vi "Result_Test.vi"(8 "error in (no error)":errorcluster caption="entrée d'erreur (pas d'erreur)", 11 "Get_Voltage en ent rée":refnum<class "Zigbee_Start_Permit_Join.lvclass">) -> (0 "error out":errorcluster caption="sortie d'erreur", 3 "Get_Voltage en sortie":refnum<class "Zigbee_Start_Permit_Join.lvclass">)   [LabVIEW 2020, in "Library Test.lvlib" / "Zigbee_Start_Permit_Join.lvclass"]
uses:
  Zigbee_Start_Permit_Join.lvclass
  C:/Users/ngarcin/OneDrive - Altyor/Standard TB/Suite TB45/Class/Test/Test (Default)/Test (Default).lvclass
  C:/Users/ngarcin/OneDrive - Altyor/Standard TB/Suite TB45/Class/Test/Zigbee_Send_Command_UART/Zigbee_Send_Command_UART.lvclass
  Commun VI/TypeDef/Variable Printable.ctl
  Zigbee_Send_Command_UART/Zigbee_Send_Command_UART.lvclass
  Commun VI/Library Commun.lvlib
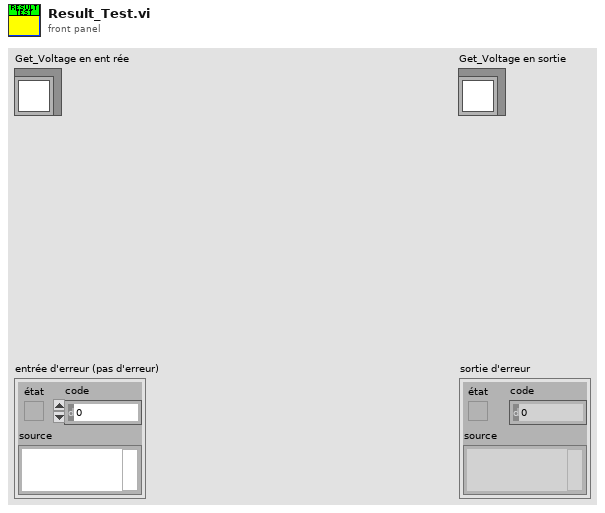
[diagram p1: front panel]
types:
  T1 = typedef "Variable Printable.ctl" = string
  T2 = enum16{"Get Variable", "Get All Variables", "Set Variable", "Delete Variable", "Delete All Variable"}
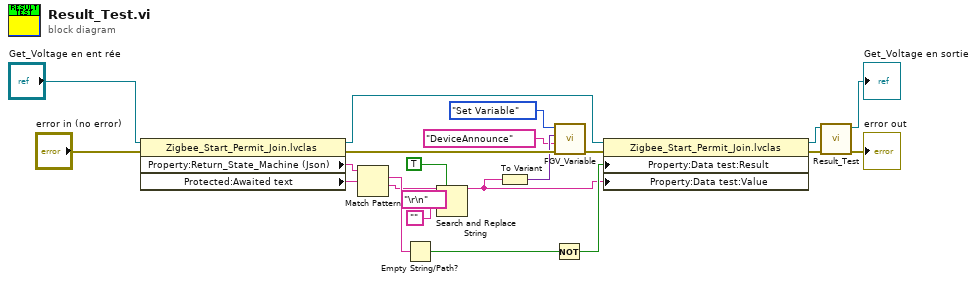
[diagram p0: block diagram]
diagram:
  n1 = property class="Zigbee_Start_Permit_Join.lvclas"(reference="Get_Voltage en ent rée", error in="error in (no error)") -> (reference out=w20:refnum<class "Zigbee_Start_Permit_Join.lvclass">, error out=w18:errorcluster, "Property:Return_State_Machine (Json)"=w17:string, "Protected:Awaited text"=w16:string)
  n2 = Match Pattern(string=w17, regular expression=w16) -> (match substring=w8:string, after substring=w4:string)  [unwired: 1 in, 2 out]
  n3 = Empty String/Path?(string/path=w8) -> (empty?=w7:bool)
  n4 = Search and Replace String(replace all?=TRUE ("tout remplacer ? (F)"), input string=w4, search string="\r\n", replace string="") -> (result string=w5:string)  [unwired: 4 in, 3 out]
  n5 = To Variant(anything=w5) -> (Variant=w15:variant)
  n6 = Not(x=w7) -> (.not. x?=w6:bool)
  n7 = call "FGV_Variable.vi"("error in (no error)"=w18, "Variable"=T1 "DeviceAnnounce", "Data In"=w15, "Function"=T2."Set Variable") -> ("error out"=w9:errorcluster)  [unwired: 5 in, 2 out]
  n8 = property class="Zigbee_Start_Permit_Join.lvclas"(reference=w20, error in=w9, "Property:Data test:Result"=w6, "Property:Data test:Value"=w5) -> (reference out=w11:refnum<class "Zigbee_Start_Permit_Join.lvclass">, error out=w12:errorcluster)
  n9 = call-parent "Result_Test.vi"("error in (no error)"=w12, "Get_Voltage en entrée"=w11) -> ("error out"=→"error out":errorcluster, "Get_Voltage en sortie"=→"Get_Voltage en sortie":refnum<class "Zigbee_Start_Permit_Join.lvclass">)  [unwired: 8 in]
